vi "Build Content.vi"(8 "error in (no error)":errorcluster, 9 "values":string[](array[string]), 10 "names":string[](array[string]), 11 "pictures":string[](array[string])) -> (0 "error out":errorcluster, 3 "<JSON>":string)   [LabVIEW 2025, in "MCP Server.lvlib"]
uses:
  MCP Server.lvlib
  199d9bb0-0593-4c5b-b65b-baf2409010c0.vi
  <vilib>/JDP Science/JSONtext/support/Format JSON Object.vi
  <vilib>/JDP Science/JSONtext/Variant to JSON Text.vi
  <vilib>/JDP Science/JSONtext/support/Format JSON Array Text.vi
  <vilib>/JDP Science/JSONtext/LVClass Serializer/JSONtext LVClass Serializer.lvclass
  <vilib>/JDP Science/JSONtext/JSONtext.lvlib
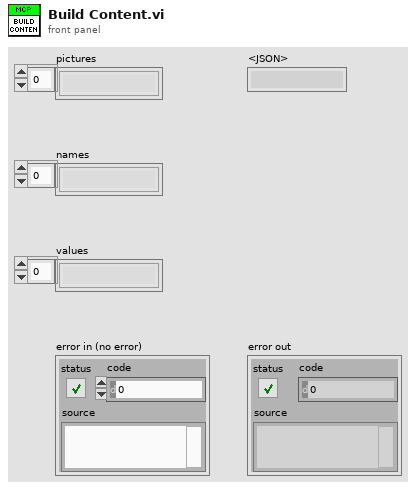
[diagram p1: front panel]
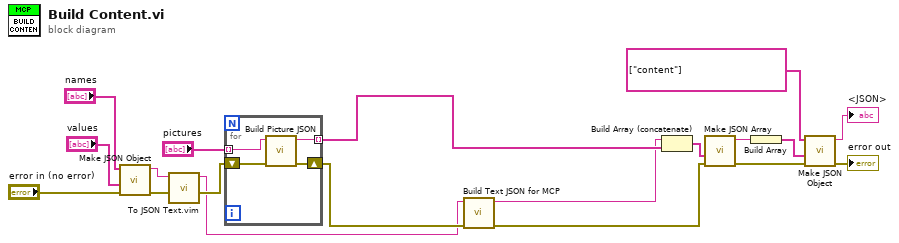
[diagram p0: block diagram]
diagram:
  n1 = call <vilib>:"Make JSON Object.vi"("error in (no error)"="error in (no error)", "JSON Items"="values", "Item Names"="names") -> ("error out"=w13:errorcluster, "<JSON>"=w8:string)  [unwired: 7 in]
  n2 = call "To JSON Text.vim"("error in (no error)"=w13, "Anything"=w8) -> ("error out"=w14:errorcluster, "<JSON>"=w9:string)  [unwired: 8 in]
  n3 = for {
    tunnel: "pictures" -> [w23] mode=indexing
    tunnel: [w22] -> w12 mode=indexing
    shift-right: [w20] -> w15
    shift-left: w14 -> [w21]
    n4 = call "Build Picture JSON.vi"("error in (no error)"=w21, "<JSON> in"=w23) -> ("error out"=w20:errorcluster, "<JSON> out"=w22:string)  [unwired: 8 in]
  }
  n5 = call "Build Text JSON for MCP.vi"("error in (no error)"=w15, "text in"=w9) -> ("error out"=w16:errorcluster, "MCP JSON text content"=w7:string)  [unwired: 8 in]
  n6 = Build Array (concatenate)(w7, w12) -> (w10:string[])
  n7 = call <vilib>:"Make JSON Array.vi"("error in (no error)"=w16, "JSON Elements"=w10) -> ("error out"=w17:errorcluster, "<JSON>"=w5:string)  [unwired: 8 in]
  n8 = Build Array(w5) -> (w6:string[])
  n9 = call <vilib>:"Make JSON Object.vi"("error in (no error)"=w17, "JSON Items"=w6, "Item Names"=string[] ["content"]) -> ("error out"=→"error out":errorcluster, "<JSON>"=→"<JSON>":string)  [unwired: 7 in]
